vi "Setup Message Channel.vi"(4 "Excluded (None)":refnum<class "Message.lvclass">[](array[class]), 6 "Included (All)":refnum<class "Message.lvclass">[](array[class]), 7 "Emit Status Messages (F)":bool, 8 "error in (no error)":errorcluster, 11 "Pub Sub Message Channel in":refnum<class "Pub Sub Message Channel.lvclass">) -> (0 "error out":errorcluster, 3 "Pub Sub Message Channel out":refnum<class "Pub Sub Message Channel.lvclass">)   [LabVIEW 2020, in "Actor Pub Sub Channels.lvlib" / "Pub Sub Message Channel.lvclass"]
uses:
  Pub Sub Message Channel.lvclass
  <vilib>/ActorFramework/Message/Message.lvclass
  Pub Sub Message Channel.lvclass/Pub Sub Message Channel.ctl
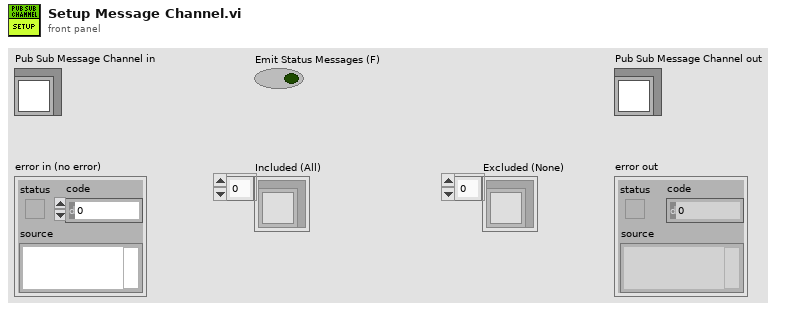
[diagram p1: front panel]
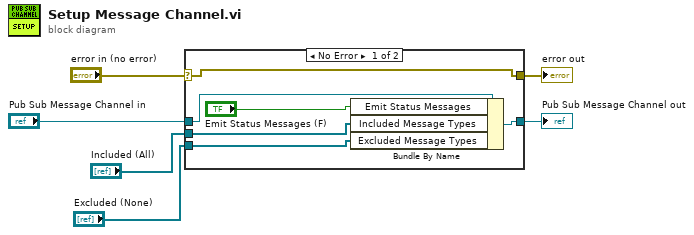
[diagram p0: block diagram]
diagram:
  n1 = case shown="No Error" "error in (no error)" {
    selector: "error in (no error)" -> [w11 w14]
    tunnel: [w11 w14] -> w5
    tunnel: [w10 w13] -> w3
    tunnel: "Pub Sub Message Channel in" -> [w12 w13]
    tunnel: "Included (All)" -> [w7 _]
    tunnel: "Excluded (None)" -> [w8 _]
    frame No Error {
      n2 = Bundle By Name(cluster=w12, "Emit Status Messages"="Emit Status Messages (F)", "Included Message Types"=w7, "Excluded Message Types"=w8) -> (w10:refnum<class "Pub Sub Message Channel.lvclass">)
    }
    frame Error {
    }
  }
  "error out" <- w5
  "Pub Sub Message Channel out" <- w3
